vi "QUIZ PROG_2.vi"() -> ()   [LabVIEW 2019]
panel:
  out "Position:CAJATop":i32
  out "Position:CLeft":i32
  out "CAJA":bool
  out "Position:Left":i32
  out "Position:Top":i32
  out "BANDA_INF":bool
  out "Valv. Negra":bool
  out "BANDA_SUP":bool
  out "Valv. Amarillo":bool
  out "Valv. Azul":bool
  out "Valv. Roja":bool
  in  "Ring":u16(ring)
  # "BODEGA"
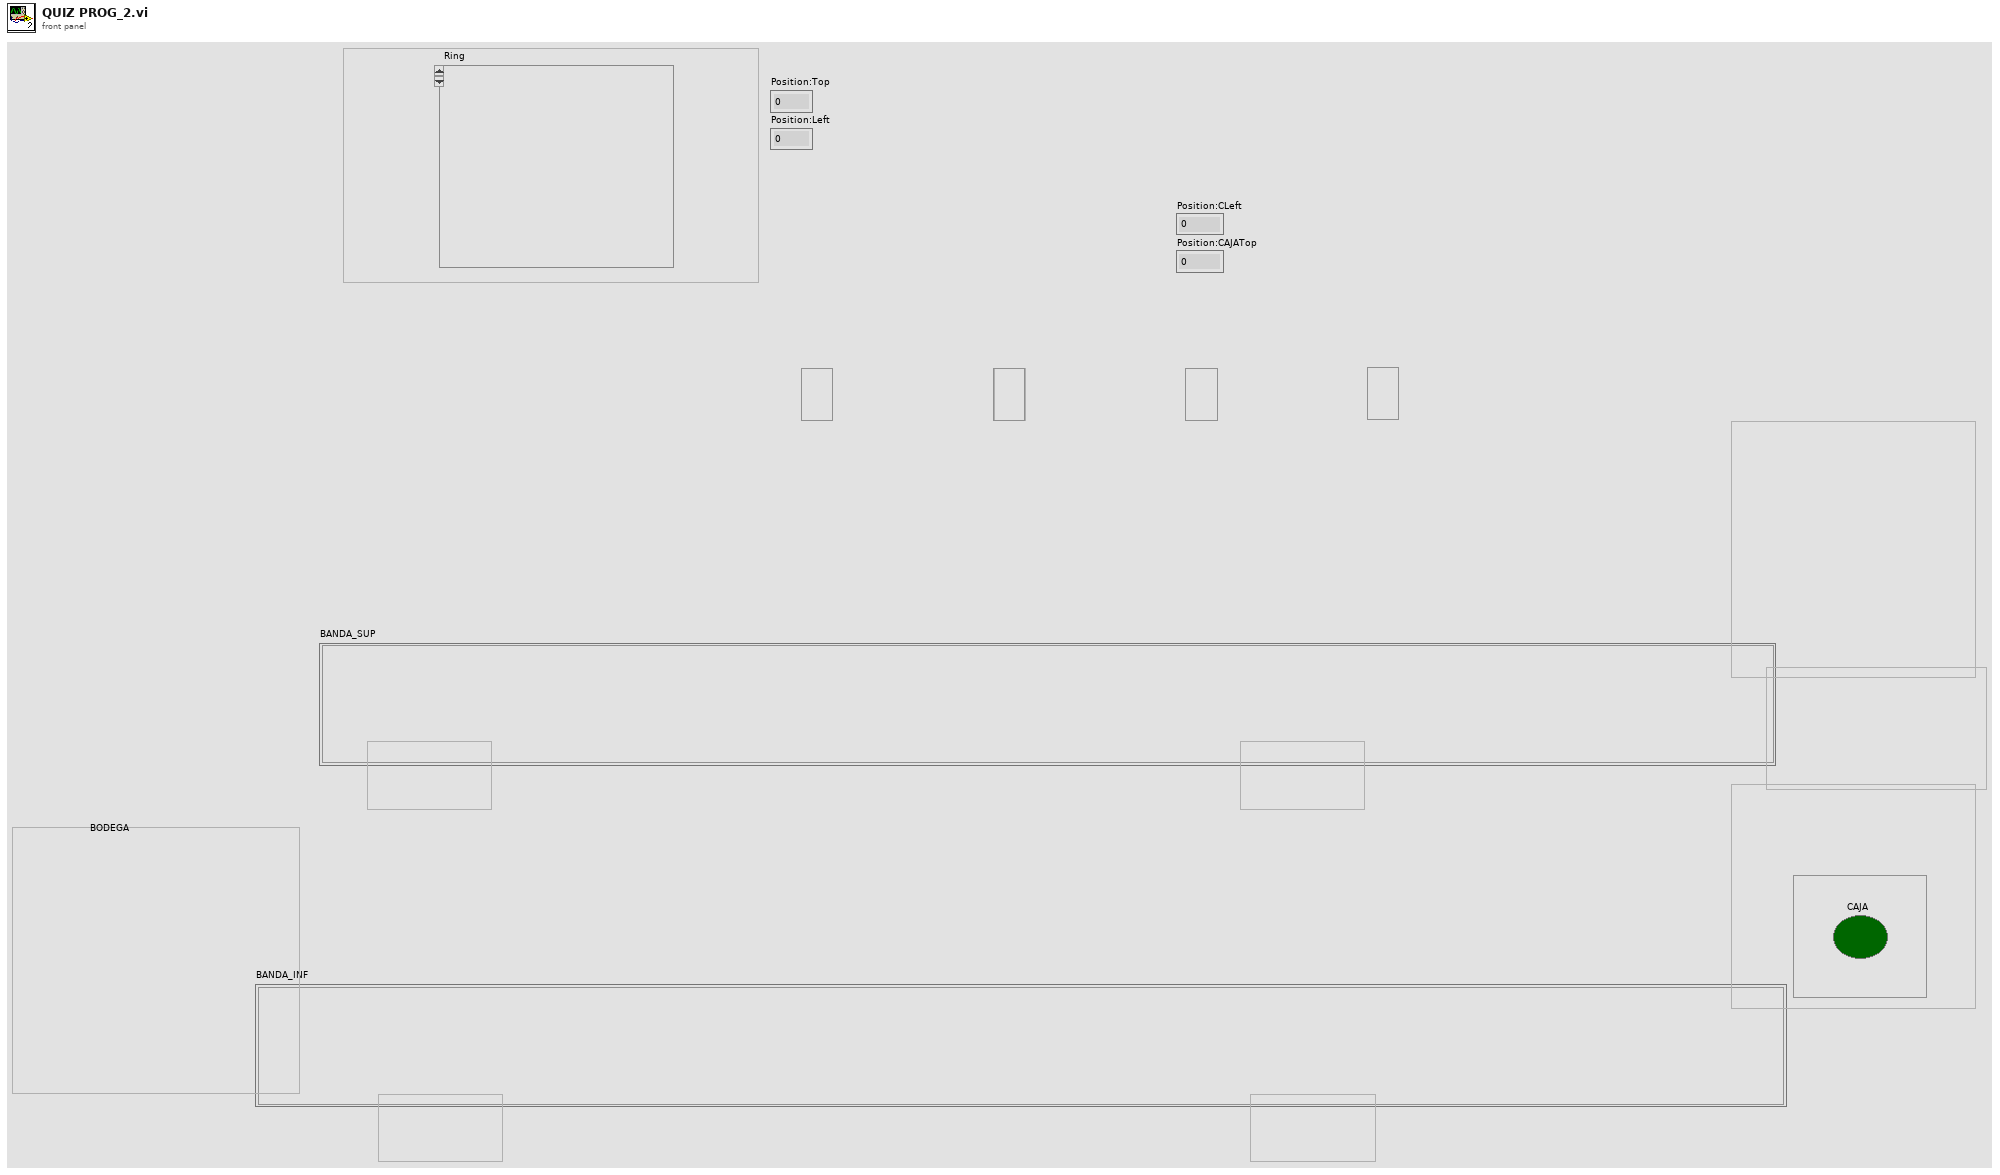
[diagram p1: front panel]
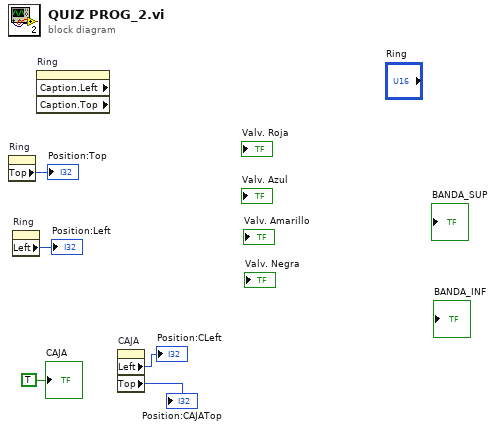
[diagram p0: block diagram]
diagram:
  n1 = property on="Ring" class="Ring (strict)"() -> ("Top"=→"Position:Top":i32)  [unwired: 2 in, 2 out]
  n2 = property on="Ring" class="Ring (strict)"() -> ("Left"=→"Position:Left":i32)  [unwired: 2 in, 2 out]
  n3 = property on="Ring" class="Ring (strict)" props=["Caption", "Left", "Caption", "Top"]() -> ()  [unwired: 2 in, 4 out]
  n4 = property on="CAJA" class="Bool (strict)"() -> ("Left"=→"Position:CLeft":i32, "Top"=→"Position:CAJATop":i32)  [unwired: 2 in, 2 out]
  "CAJA" <- TRUE ("CAJA")
